vi "Main.vi"() -> ()   [LabVIEW 2018]
panel:
  out "concatenated string":string
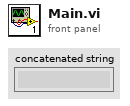
[diagram p1: front panel]
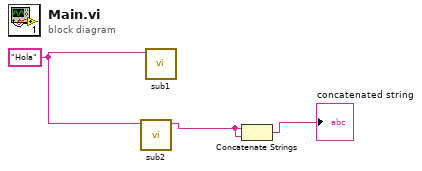
[diagram p0: block diagram]
diagram:
  w3 = "Hola"
  n1 = call "sub2.vi"("String in"=w3) -> ("String out"=w1:string)  [unwired: 10 in]
  n2 = call "sub1.vi"("String"=w3) -> ()  [unwired: 11 in]
  n3 = Concatenate Strings(w1, w1) -> (→"concatenated string":string)
